vi "LoadVIsFromProject.vi"(8 "error in (no error)":errorcluster, 11 "ProjectPath":path) -> (0 "error out":errorcluster, 2 "Project":refnum<vi>, 3 "VIs":refnum<vi>[](array[refnum]))   [LabVIEW 2020]
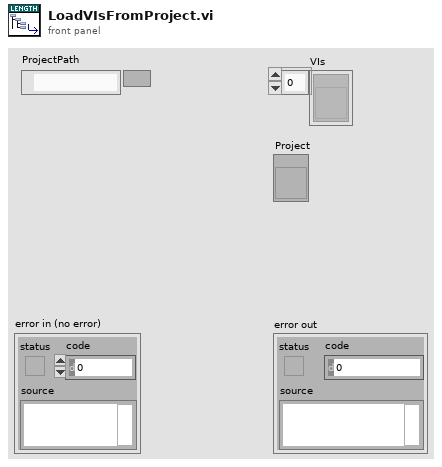
[diagram p1: front panel]
types:
  T1 = enum32{"invalid VI type", "Standard VI", "Control VI", "Global VI", "Polymorphic VI", "Configuration VI", "SubSystem", "Facade VI", "Method VI", "Statechart Diagram VI"}
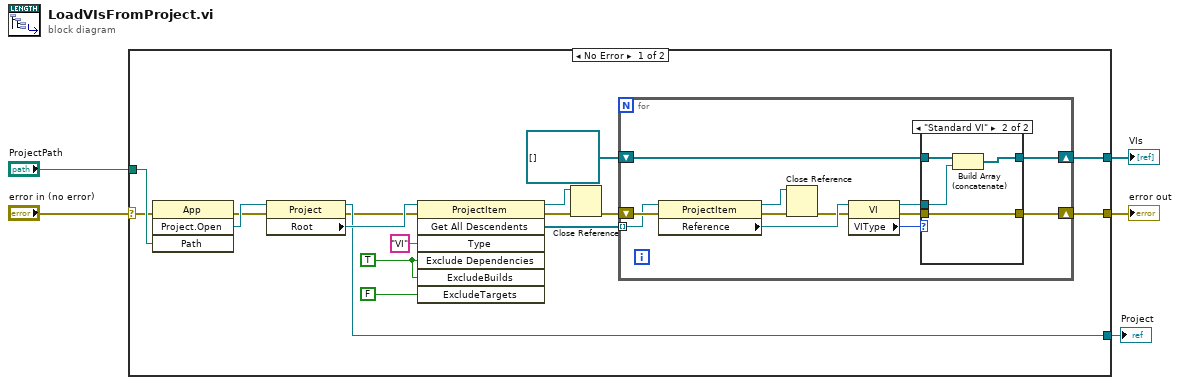
[diagram p0: block diagram]
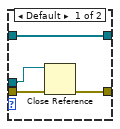
[diagram p2: hidden frame]
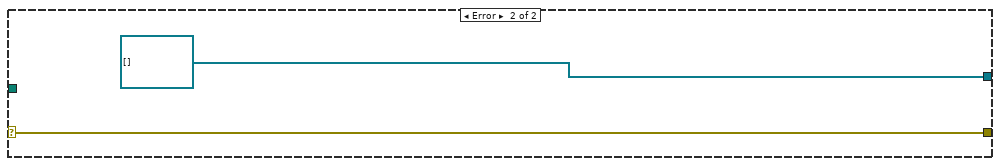
[diagram p3: hidden frame]
diagram:
  n1 = case shown="No Error" "error in (no error)" {
    selector: "error in (no error)" -> [w21 w44]
    tunnel: [w11 w44] -> w5
    tunnel: "ProjectPath" -> [w22 _]
    tunnel: [w12 refnum<vi>[] []] -> w2
    tunnel: [w7 _] -> w1
    frame No Error {
      w9 = TRUE ("ExcludeDependencies")
      n2 = invoke class="App" method="Project.Open"(error in=w21, "Path"=w22) -> (error out=w19:errorcluster, "Project:Open"=w20:refnum<vi>)  [unwired: 2 in, 2 out]
      n3 = property class="Project"(reference=w20, error in=w19) -> (reference out=w7:refnum<vi>, error out=w6:errorcluster, "Root"=w18:refnum<vi>)
      n4 = invoke class="ProjectItem" method="Get All Descendents"(reference=w18, error in=w6, "Type"="VI", "Exclude Dependencies"=w9, "ExcludeBuilds"=w9, "ExcludeTargets"=FALSE) -> (reference out=w10:refnum<vi>, error out=w15:errorcluster, "All Descendents"=w16:refnum<vi>[])  [unwired: 1 in, 4 out]
      n5 = Close Reference(reference=w10, error in (no error)=w15) -> (error out=w14:errorcluster)
      n6 = for {
        tunnel: w16 -> [w33] mode=indexing
        shift-right: [w25] -> w11
        shift-left: w14 -> [w34]
        shift-right: [w24] -> w12
        shift-left: refnum<vi>[] [] -> [w23]
        n7 = property class="ProjectItem"(reference=w33, error in=w34) -> (reference out=w31:refnum<vi>, error out=w32:errorcluster, "Reference"=w30:refnum<vi>)
        n8 = Close Reference(reference=w31, error in (no error)=w32) -> (error out=w29:errorcluster)
        n9 = property class="VI"(reference=w30, error in=w29) -> (reference out=w26:refnum<vi>, error out=w27:errorcluster, "VIType"=w28:T1)
        n10 = case shown="\"Standard VI\"" w28 {
          tunnel: w27 -> [w38 w42]
          tunnel: w26 -> [w36 w41]
          tunnel: [w37 w42] -> w25
          tunnel: [w35 w40] -> w24
          tunnel: w23 -> [w35 w39]
          frame Default {
            n11 = Close Reference(reference=w36, error in (no error)=w38) -> (error out=w37:errorcluster)
          }
          frame "Standard VI" {
            n12 = Build Array (concatenate)(w39, w41) -> (w40:refnum<vi>[])
          }
        }
      }
    }
    frame Error {
    }
  }
  "error out" <- w5
  "VIs" <- w2
  "Project" <- w1
